vi "Count Pairs.vi"(6 "Amount":i64, 7 "Pair":string, 11 "Pair Map In":map{string, i64}(c390)) -> (3 "Pair Map Out":map{string, i64}(c390))   [LabVIEW 2021]
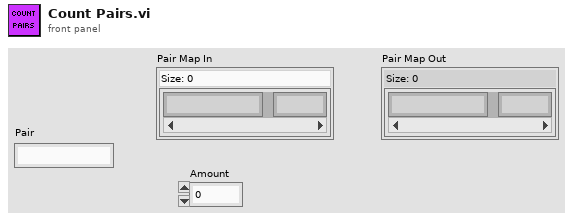
[diagram p1: front panel]
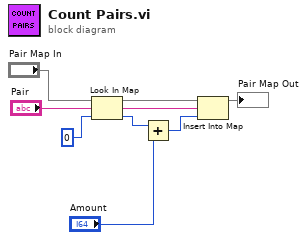
[diagram p0: block diagram]
diagram:
  n1 = Look In Map(map="Pair Map In", key="Pair", default value=0) -> (value=w2:i64)  [unwired: 1 out]
  n2 = Add(x=w2, y="Amount") -> (x+y=w5:i64)
  n3 = Insert Into Map(map in="Pair Map In", key="Pair", value=w5) -> (map out=→"Pair Map Out":map{string, i64})  [unwired: 2 out]
